vi "reshape.channels.vi"(9 "y.pixels":dbl, 10 "x.pixels":dbl, 11 "element":dbl[][](array[numeric])) -> (3 "Array":dbl[][][](array[numeric]))   [LabVIEW 2017]
doc: "SciScan 1.2 160622"
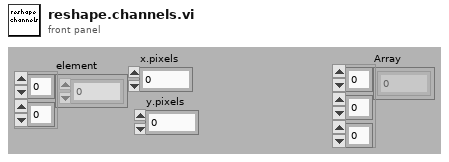
[diagram p1: front panel]
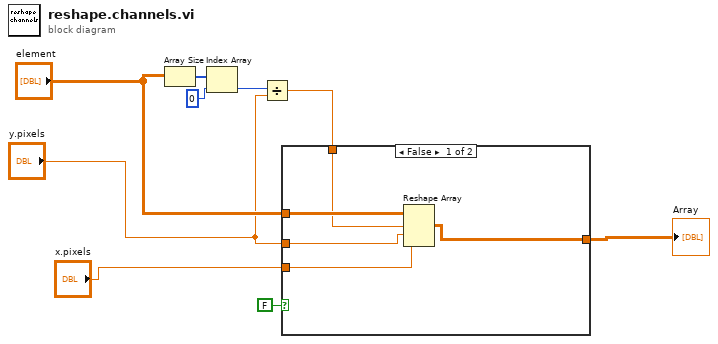
[diagram p0: block diagram]
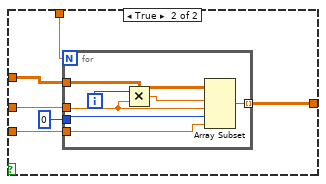
[diagram p2: hidden frame]
diagram:
  n1 = Array Size(array="element") -> (size(s)=w8:i32[])
  n2 = Index Array(array=w8, index=0) -> (element=w6:i32)
  n3 = Divide(x=w6, y="y.pixels") -> (x/y=w5:dbl)
  n4 = case shown="False" FALSE {
    tunnel: "element" -> [w14 w19]
    tunnel: w5 -> [w13 w18]
    tunnel: [w10 w17] -> w4
    tunnel: "y.pixels" -> [w12 w16]
    tunnel: "x.pixels" -> [w11 w15]
    frame False {
      n5 = Reshape Array(w14, w13, w12, w11) -> (w10:dbl[][][])
    }
    frame True {
      n6 = for {
        N: w18 -> [_]
        tunnel: w19 -> [w27]
        tunnel: w15 -> [w26]
        tunnel: 0 ("index") -> [w25]
        tunnel: w16 -> [w23]
        tunnel: [w21] -> w17 mode=indexing
        i -> [w24]
        n7 = Multiply(x=w24, y=w23) -> (x*y=w22:dbl)
        n8 = Array Subset(array=w27, index (row)=w22, length (row)=w23, index (col)=w25, length (col)=w26) -> (w21:dbl[][])
      }
    }
  }
  "Array" <- w4
